vi "Enqueue Test.vi"(8 "error in (no error)":errorcluster, 10 "Test to Enqueue":refnum<class "Test.lvclass">, 11 "Test Manager in":refnum<class "Test Manager.lvclass">) -> (0 "error out":errorcluster, 3 "Test Manager out":refnum<class "Test Manager.lvclass">)   [LabVIEW 2020, in "Test Manager.lvlib" / "Test Manager.lvclass"]
uses:
  Test Manager.lvclass
  _Abstract Classes/Test/Test.lvclass
  Test Manager.lvclass/Test Manager.ctl
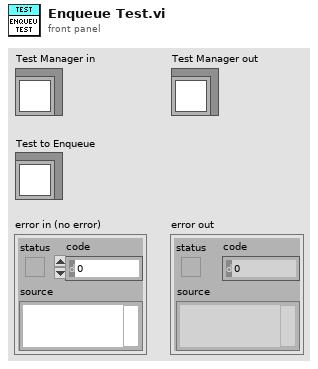
[diagram p1: front panel]
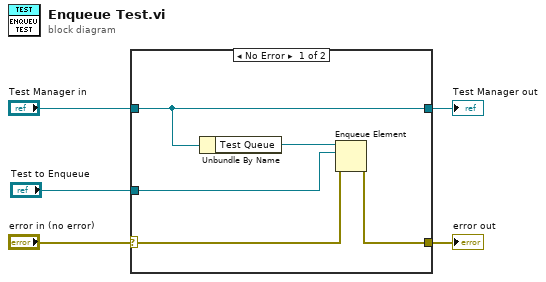
[diagram p0: block diagram]
diagram:
  n1 = case shown="No Error" "error in (no error)" {
    selector: "error in (no error)" -> [w8 w12]
    tunnel: [w7 w12] -> w4
    tunnel: [w10 w11] -> w2
    tunnel: "Test Manager in" -> [w10 w11]
    tunnel: "Test to Enqueue" -> [w6 _]
    frame No Error {
      n2 = Unbundle By Name(w10) -> ("Test Queue"=w9:refnum<queue>)
      n3 = Enqueue Element(queue=w9, element=w6, error in (no error)=w8) -> (error out=w7:errorcluster)  [unwired: 1 in, 2 out]
    }
    frame Error {
    }
  }
  "error out" <- w4
  "Test Manager out" <- w2
